vi "Find_Puck_And_Players (tidy).vi"(6 "Puck and Player Settings":T2={"Noise Erosion"=10, "Find Circles (Min Radius)"=20.0, "Find Circles (Max Radius)"=50.0, "Cutoff Radius  "=34.0}, 8 "Error In":errorcluster, 10 "ROI Descriptor (Tab) in":T3 {"Contours"."Type" items=["No Selection", "Point", "Line", "Rectangle", "Oval", "Polygon", "Freehand Region", "Annulus", "Unused2", "Unused3", "Broken Line", "Freehand Line", "Rotated Rectangle"]}, 11 "Image In":T1) -> (0 "Error Out":errorcluster, 1 "Puck and Player Position":T4)   [LabVIEW 2017]
uses:
  <vilib>/vision/Image Controls.llb/IMAQ Image.ctl
  <vilib>/vision/NI_Vision_Development_Module.lvlib
panel:
  out "Image Out":T1
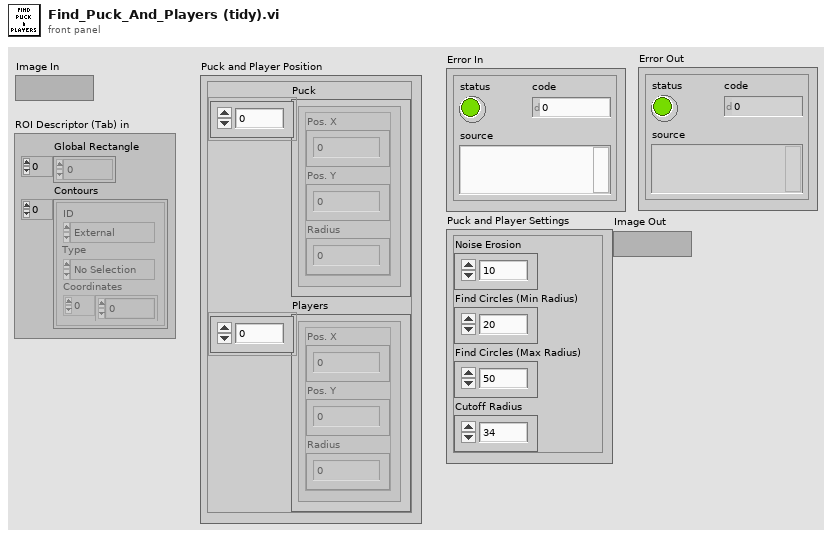
[diagram p1: front panel]
types:
  T1 = typedef "IMAQ Image.ctl" = refnum<image>
  T2 = cluster{"Noise Erosion":i32, "Find Circles (Min Radius)":sgl, "Find Circles (Max Radius)":sgl, "Cutoff Radius  ":sgl}
  T3 = typedef "ROI Descriptor" = cluster{"Global Rectangle":i32[], "Contours":cluster{"ID":enum32{"External", "Internal"}, "Type":u32, "Coordinates":i32[]}[]}
  T4 = cluster{"Puck":cluster{"Pos. X":i32, "Pos. Y":i32, "Radius":i32}[], "Players":cluster{"Pos. X":i32, "Pos. Y":i32, "Radius":i32}[]}
  T5 = cluster{"Pos. X":i32, "Pos. Y":i32, "Radius":i32, "Core Area":i32}[]
  T6 = cluster{"Pos. X":i32, "Pos. Y":i32, "Radius":i32, "Core Area":i32}
  T7 = cluster{"Pos. X":i32, "Pos. Y":i32, "Radius":i32}[]
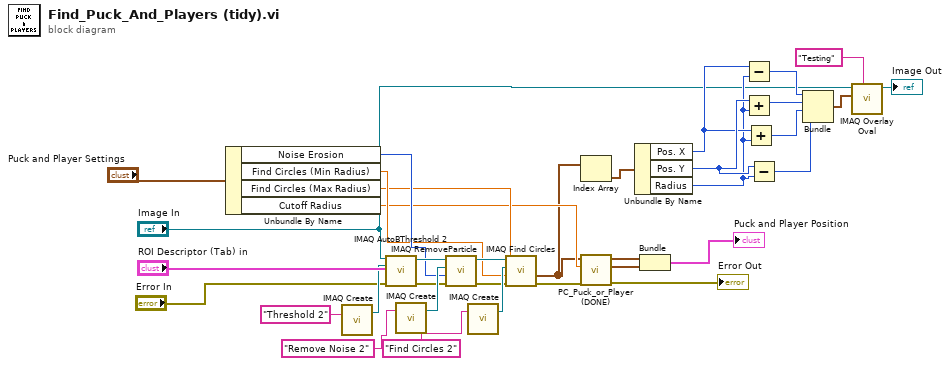
[diagram p0: block diagram]
diagram:
  n1 = Unbundle By Name("Puck and Player Settings") -> ("Noise Erosion"=w17:i32, "Find Circles (Min Radius)"=w16:sgl, "Find Circles (Max Radius)"=w15:sgl, "Cutoff Radius"=w14:sgl)
  n2 = call "IMAQ Create"("Image Name"="Threshold 2") -> ("New Image"=w20:T1)  [unwired: 4 in, 1 out]
  n3 = call "IMAQ AutoBThreshold 2"("Image Src"="Image In", "Image Dst"=w20, "ROI Descriptor"="ROI Descriptor (Tab) in", "error in (no error)"="Error In") -> ("Image Dst Out"=w22:T1, "error out"=w21:errorcluster)  [unwired: 9 in, 1 out]
  n4 = call "IMAQ Create"("Image Name"="Remove Noise 2") -> ("New Image"=w23:T1)  [unwired: 4 in, 1 out]
  n5 = call "IMAQ RemoveParticle"("error in (no error)"=w21, "Number of Erosion"=w17, "Image Dst"=w23, "Image Src"=w22) -> ("error out"=w25:errorcluster, "Image Dst Out"=w26:T1)  [unwired: 6 in]
  n6 = call "IMAQ Create"("Image Name"="Find Circles 2") -> ("New Image"=w27:T1)  [unwired: 4 in, 1 out]
  n7 = call "IMAQ Find Circles"("Max Radius"=w15, "error in (no error)"=w25, "Min Radius"=w16, "Image Dst"=w27, "Image Src"=w26) -> ("error out"=w24:errorcluster, "Circles Data"=w13:T5)  [unwired: 3 in, 2 out]
  n8 = Index Array(array=w13) -> (element=w12:T6)  [unwired: 1 in]
  n9 = call "PC_Puck_or_Player (DONE).vi"("Error In"=w24, "Cutoff"=w14, "Circles Data"=w13) -> ("Error Out"=→"Error Out":errorcluster, "Players"=w30:T7, "Puck"=w29:T7)  [unwired: 6 in]
  n10 = Unbundle By Name(w12) -> ("Pos. X"=w10:i32, "Pos. Y"=w11:i32, "Radius"=w9:i32)
  n11 = Bundle("Puck"=w29, "Players"=w30) -> (→"Puck and Player Position":T4)  [unwired: 1 in]
  n12 = Subtract(x=w10, y=w9) -> (x-y=w8:i32)
  n13 = Add(x=w11, y=w9) -> (x+y=w7:i32)
  n14 = Add(x=w10, y=w9) -> (x+y=w6:i32)
  n15 = Subtract(x=w11, y=w9) -> (x-y=w5:i32)
  n16 = Bundle(w8, w7, w6, w5) -> (w4:cluster{i32, i32, i32, i32})  [unwired: 1 in]
  n17 = call "IMAQ Overlay Oval"("Group"="Testing", "Bounding Rectangle"=w4, "Image"="Image In") -> ("Image Out"=→"Image Out":T1)  [unwired: 7 in, 1 out]
